vi "Parse HTTP Return Code.vi"(11 "headers":string) -> (1 "message":string, 2 "code":i32, 3 "protocol":string)   [LabVIEW 2014, in "Raspberry Pi Compatible Compiler for LabVIEW.lvlib" / "GitHub API.lvlib"]
uses:
  GitHub API.lvlib
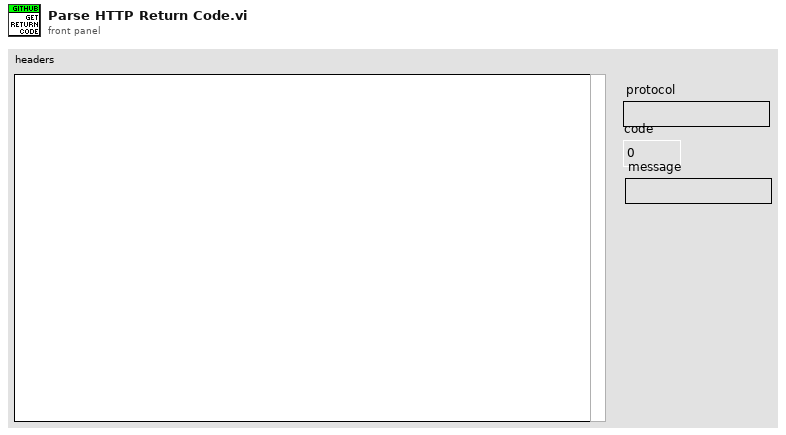
[diagram p1: front panel]
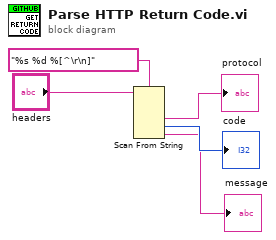
[diagram p0: block diagram]
diagram:
  n1 = Scan From String(format string="%s %d %[^\r\n]", input string="headers") -> (output 1=→"protocol":string, output 2=→"code":i32, output 3=→"message":string)  [unwired: 5 in, 3 out]
